vi "FRC Gyro and Accel Example.vi"() -> ()   [LabVIEW 2015]
doc: "SimpleGyro Example\n\nThis example shows how to use a SimpleGyro sensor connected to the SPI port on the RoboRIO.\n\nThis example expects a USB cable connected from your development PC to the Type B USB Jack (next to the power input) on the roboRIO."
uses:
  <vilib>/Rock Robotics/SystemInterfaces/spilib/spi_bus.ctl
  SimpleGyro/FRC Gyro and Accel.lvlib
panel:
  out "Finished Calibrating?":bool
  in  "Reset Angle?":bool
  out "Device Found":bool
  in  "stop":bool
  out "Angle":dbl(knob) scale=0.0..360.0
  in  "SPI Chip Select":T1
  in  "Sample Rate (ms)":dbl=1.0 min=0.0 max=100.0 step=0.25 format="%#_13g"
  # "FRC Gyro & Accel Example"
  # "Gyro Configuration \n(Can Only Be Changed at Start-Up)"
  # "FRC Gyro & Accel Placement"
  # "How to Install the FRC Gyro & Accel"
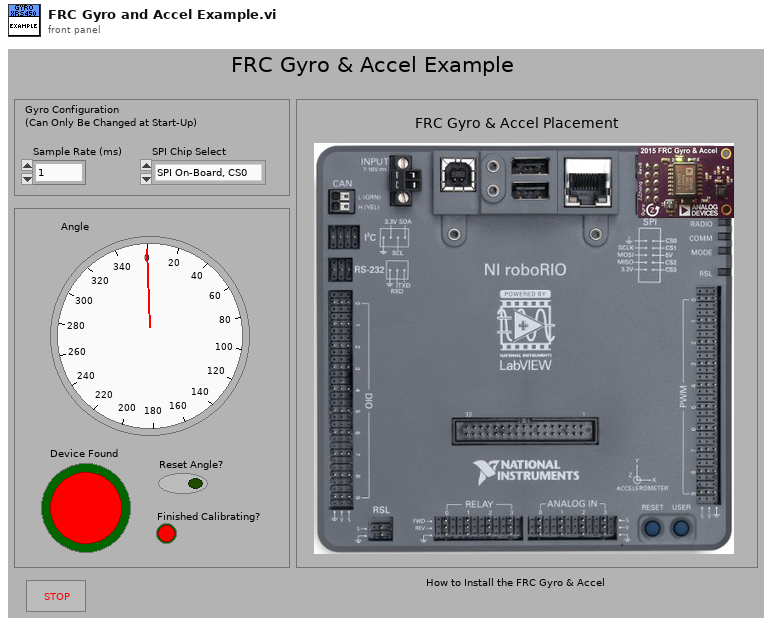
[diagram p1: front panel]
types:
  T1 = typedef "spi_bus.ctl" = enum16{"SPI On-Board, CS0", "SPI On-Board, CS1", "SPI On-Board, CS2", "SPI On-Board, CS3", "SPI MXP", "Invalid"}
  T2 = typedef "FRC Gyro and Accel.lvlib/WPI_SimpleGyroDevRef.ctl" = cluster{"DevStatus":errorcluster, "Handle":i32, "SPI Bus":T1, "Device Found":bool, "Sample Rate":dbl}
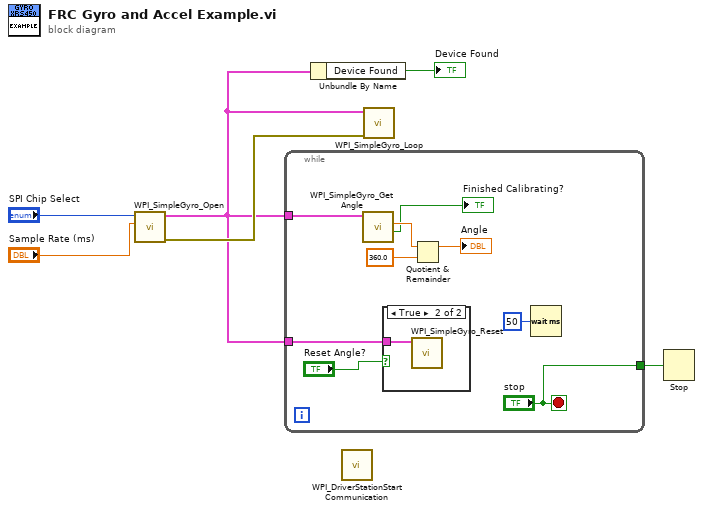
[diagram p0: block diagram]
diagram:
  n1 = call "WPI_SimpleGyro_Open.vi"("Sample Rate (ms)"="Sample Rate (ms)", "SPI Chip Select"="SPI Chip Select") -> ("error out"=w6:errorcluster, "SimpleGyroDevRef"=w1:T2)  [unwired: 8 in]
  n2 = while {
    tunnel: w1 -> [w8]
    tunnel: ["stop"] -> w3
    tunnel: w1 -> [w10]
    stop <- "stop" stop-if-true
    n3 = call "WPI_SimpleGyro_Get Angle.vi"("SimpleGyroDevRef"=w8) -> ("Calibrated?"=→"Finished Calibrating?":bool, "Angle"=w15:dbl)  [unwired: 7 in, 2 out]
    n4 = case shown="True" "Reset Angle?" {
      tunnel: w10 -> [_ w16]
      frame False {
      }
      frame True {
        n5 = call "WPI_SimpleGyro_Reset.vi"("SimpleGyroDevRef"=w16) -> ()  [unwired: 9 in, 2 out]
      }
    }
    n6 = Quotient & Remainder(x=w15, y=360.0) -> (x-y*floor(x/y)=→"Angle":dbl)  [unwired: 1 out]
    n7 = Wait (ms)(milliseconds to wait=u32 50) -> ()  [unwired: 1 out]
  }
  n8 = Unbundle By Name(w1) -> ("Device Found"=→"Device Found":bool)
  n9 = call <vilib>:"WPI_DriverStationStart Communication.vi"() -> ()  [unwired: 12 in]
  n10 = call "WPI_SimpleGyro_Loop.vi"("error in"=w6, "SimpleGyroDevRef"=w1) -> ()  [unwired: 9 in, 1 out]
  n11 = Stop(stop? (T)=w3) -> ()
